vi "Read irqNumber.vi"(8 "error in (no error)":errorcluster, 11 "IRQConfig in":refnum<class "IRQConfig.lvclass">) -> (0 "error out":errorcluster, 2 "irqNumber":i32, 3 "IRQConfig out":refnum<class "IRQConfig.lvclass">)   [LabVIEW 2013, in "ComponentData.lvlib" / "IRQConfig.lvclass"]
uses:
  <userlib>/Common/Component/Application/RT/ComponentData/ConfigurationHandler/IRQConfig/IRQConfig.lvclass
  <userlib>/Common/Component/Application/RT/ComponentData/ConfigurationHandler/IRQConfig/IRQConfig.lvclass/IRQConfig.ctl
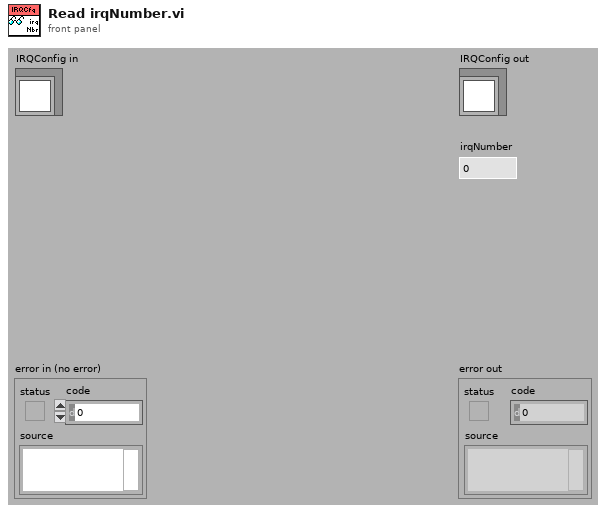
[diagram p1: front panel]
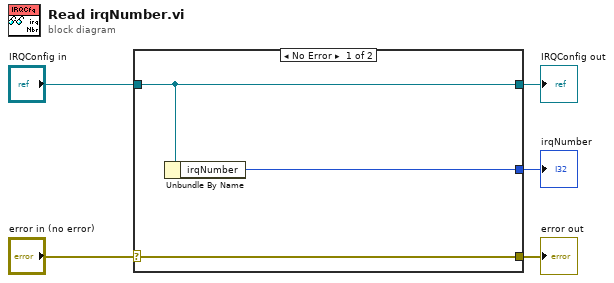
[diagram p0: block diagram]
diagram:
  n1 = case shown="No Error" "error in (no error)" {
    selector: "error in (no error)" -> [w8 w9]
    tunnel: [w8 w9] -> w4
    tunnel: [w7 w10] -> w2
    tunnel: "IRQConfig in" -> [w7 w10]
    tunnel: [w6 _] -> w1
    frame No Error {
      n2 = Unbundle By Name(w7) -> ("irqNumber"=w6:i32)
    }
    frame Error {
    }
  }
  "error out" <- w4
  "IRQConfig out" <- w2
  "irqNumber" <- w1
